vi "Place application on Desktop position.vi"(4 "Fragmental Window name":string="Hamlib Rotorctld") -> ()   [LabVIEW 2013]
panel:
  out "Übereinstimmender Teil-String":string
  in  "OpenVIs":bool
  out "All Windows":string[](array[string])
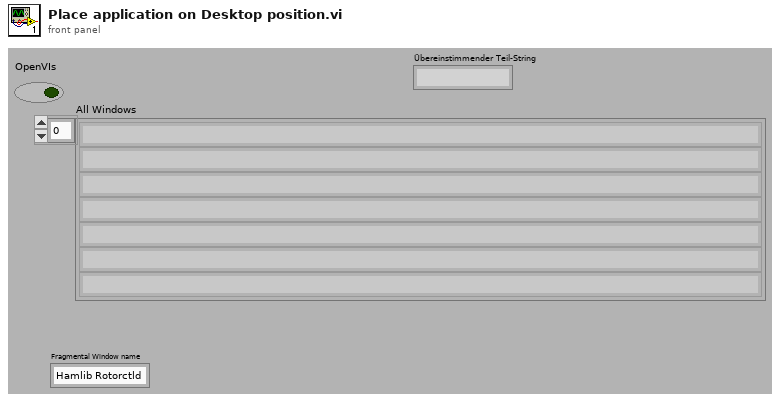
[diagram p1: front panel]
types:
  T1 = typedef "Window Refnum.ctl" = refnum<k1>
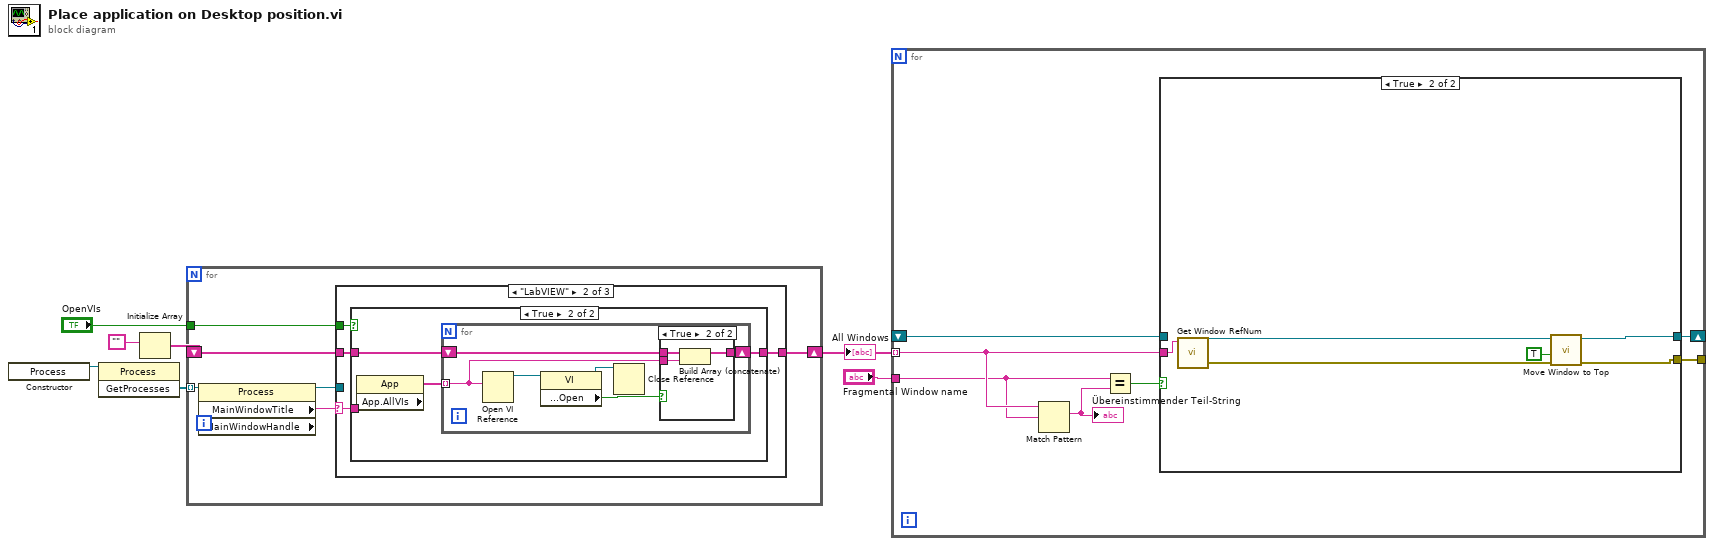
[diagram p0: block diagram]
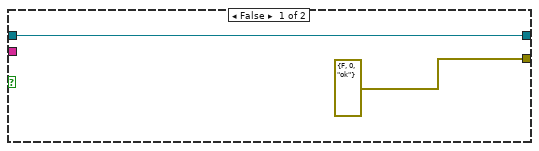
[diagram p2: hidden frame]
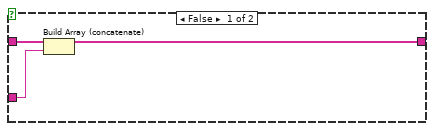
[diagram p4: hidden frame]
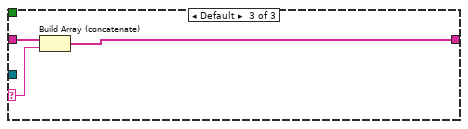
[diagram p6: hidden frame]
diagram:
  n1 = constructor class="Process"() -> (reference out=w7:refnum<k24>)  [unwired: 3 in, 2 out]
  n2 = invoke class="Process" method="GetProcesses"(reference=w7) -> ("GetProcesses"=w6:refnum<k24>[])  [unwired: 2 in, 2 out]
  n3 = Initialize Array("") -> (w5:string[])  [unwired: 1 in]
  n4 = for {
    tunnel: w6 -> [w9] mode=indexing
    shift-right: [w12] -> w2
    shift-left: w5 -> [w13]
    tunnel: "OpenVIs" -> [w8]
    n5 = property class="Process" props=["MainWindowTitle", "MainWindowHandle"](reference=w9) -> (reference out=w11:refnum<k24>, "MainWindowTitle"=w10:string)  [unwired: 1 in, 2 out]
    n6 = case shown="\"LabVIEW\"" w10 {
      selector: w10 -> [_ w15 w35]
      tunnel: w13 -> [w14 w18 w37]
      tunnel: [w14 w17 w36] -> w12
      tunnel: w11 -> [_ _ _]
      tunnel: w8 -> [_ w16 _]
      frame "" {
      }
      frame "LabVIEW" {
        n7 = case shown="True" w16 {
          tunnel: w18 -> [w21 w23]
          tunnel: [w19 w22] -> w17
          tunnel: w15 -> [w20 _]
          frame False {
            n8 = Build Array (concatenate)(w21, w20) -> (w19:string[])
          }
          frame True {
            n9 = property class="App"() -> ("App.AllVIs"=w24:string[])  [unwired: 2 in, 2 out]
            n10 = for {
              tunnel: w24 -> [w28] mode=indexing
              shift-right: [w27] -> w22
              shift-left: w23 -> [w29]
              n11 = Open VI Reference(vi path=w28) -> (vi reference=w30:refnum<vi>)  [unwired: 5 in, 1 out]
              n12 = property class="VI"(reference=w30) -> (reference out=w25:refnum<vi>, "Front Panel.Open"=w26:bool)  [unwired: 1 in, 1 out]
              n13 = Close Reference(reference=w25) -> ()  [unwired: 1 in, 1 out]
              n14 = case shown="True" w26 {
                tunnel: w29 -> [w31 w34]
                tunnel: w28 -> [_ w33]
                tunnel: [w31 w32] -> w27
                frame False {
                }
                frame True {
                  n15 = Build Array (concatenate)(w34, w33) -> (w32:string[])
                }
              }
            }
          }
        }
      }
      frame Default {
        n16 = Build Array (concatenate)(w37, w35) -> (w36:string[])
      }
    }
  }
  "All Windows" <- w2
  n17 = for {
    tunnel: w2 -> [w43] mode=indexing
    tunnel: [w41] -> _
    tunnel: "Fragmental Window name" -> [w40]
    shift-right: [w39] -> _
    shift-left: _ -> [w38]
    n18 = Match Pattern(string=w43, regular expression=w40) -> (match substring=w44:string)  [unwired: 1 in, 3 out]
    "Übereinstimmender Teil-String" <- w44
    n19 = Equal?(x=w40, y=w44) -> (x = y?=w42:bool)
    n20 = case shown="True" w42 {
      tunnel: w43 -> [_ w52]
      tunnel: [errorcluster {"status"=FALSE, "code"=0, "source"="ok"} ("error out") w51] -> w41
      tunnel: [w45 w50] -> w39
      tunnel: w38 -> [w45 _]
      frame False {
      }
      frame True {
        n21 = call "Get Window RefNum.vi"("window name (\"\")"=w52) -> ("error out"=w48:errorcluster, "window refnum (NaWR)"=w49:T1)  [unwired: 7 in]
        n22 = call "Move Window to Top.vi"("error in (no error)"=w48, "activate? (T)"=TRUE, "window refnum (NaWR)"=w49) -> ("error out"=w51:errorcluster, "window refnum out"=w50:T1)  [unwired: 3 in]
      }
    }
  }
